vi "CalculateLuhnNumber.vi"(10 "InputString":string) -> (2 "String 2":string, 4 "Valid":bool)   [LabVIEW 2022 SP3]
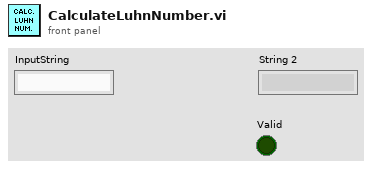
[diagram p1: front panel]
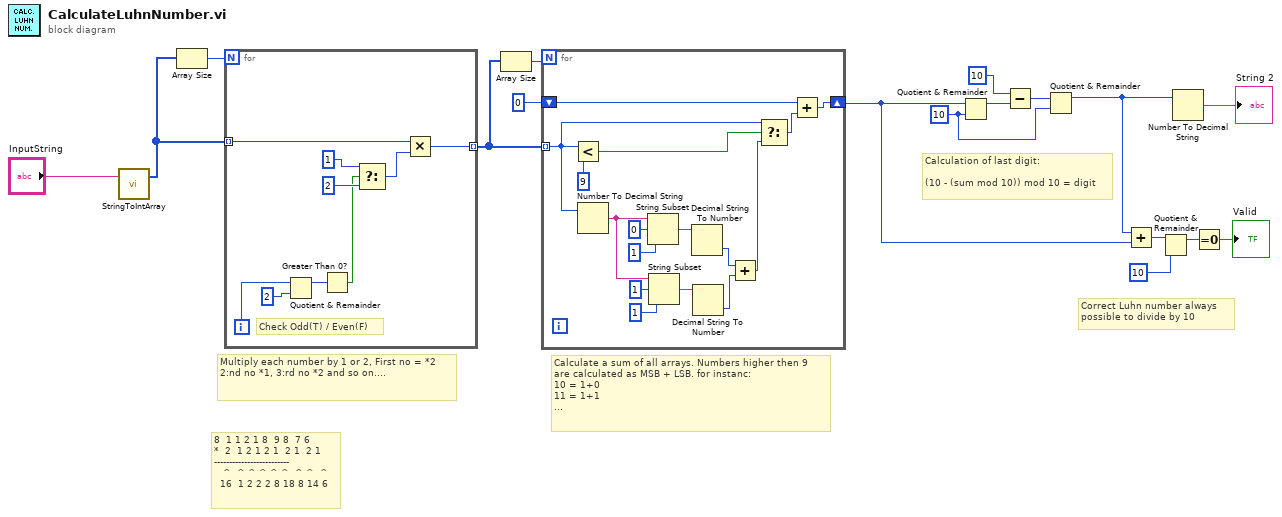
[diagram p0: block diagram]
diagram:
  w7 = 10 ("y")
  # "Correct Luhn number always\npossible to divide by 10"
  # "Calculation of last digit:\n\n(10 - (sum mod 10)) mod 10 = digit"
  # "8  1 1 2 1 8  9 8  7 6\n*  2  1 2 1 2 1  2 1  2 1\n-------------------------\n   ^  ^ ^ ^ ^ ^  ^ ^  ^ \n  16  1 2 2 2 8 18 8 14 6"
  # "Calculate a sum of all arrays. Numbers higher then 9\nare calculated as MSB + LSB. for instanc:\n10 = 1+0\n11 = 1+1\n..."
  # "Multiply each number by 1 or 2, First no = *2\n2:nd no *1, 3:rd no *2 and so on...."
  n1 = call "StringToIntArray.vi"("InputString"="InputString") -> ("OutArray"=w15:i32[])  [unwired: 1 in, 1 out]
  n2 = Array Size(array=w15) -> (size(s)=w16:i32)
  n3 = for {
    N: w16 -> [_]
    tunnel: w15 -> [w23] mode=indexing
    tunnel: [w18] -> w13 mode=indexing
    i -> [w24]
    # "Check Odd(T) / Even(F)"
    n4 = Quotient & Remainder(x=w24, y=2) -> (x-y*floor(x/y)=w26:i32)  [unwired: 1 out]
    n5 = Greater Than 0?(x=w26) -> (x > 0?=w19:bool)
    n6 = Select(t=1, s=w19, f=2) -> (s? t:f=w22:i32)
    n7 = Multiply(x=w23, y=w22) -> (x*y=w18:i32)
  }
  n8 = Array Size(array=w13) -> (size(s)=w14:i32)
  n9 = for {
    N: w14 -> [_]
    tunnel: w13 -> [w37] mode=indexing
    shift-right: [w41] -> w5
    shift-left: 0 -> [w39]
    n10 = Less?(x=w37, y=9) -> (x < y?=w40:bool)
    n11 = Number To Decimal String(number=w37) -> (decimal integer string=w30:string)  [unwired: 1 in]
    n12 = String Subset(string=w30, offset (0)=0, length (rest)=1 ("length (rest)")) -> (substring=w34:string)
    n13 = String Subset(string=w30, offset (0)=1, length (rest)=1 ("length (rest)")) -> (substring=w31:string)
    n14 = Decimal String To Number(string=w34) -> (number=w29:i32)  [unwired: 2 in, 1 out]
    n15 = Decimal String To Number(string=w31) -> (number=w28:i32)  [unwired: 2 in, 1 out]
    n16 = Add(x=w29, y=w28) -> (x+y=w27:i32)
    n17 = Select(t=w37, s=w40, f=w27) -> (s? t:f=w38:i32)
    n18 = Add(x=w39, y=w38) -> (x+y=w41:i32)
  }
  n19 = Quotient & Remainder(x=w5, y=w7) -> (x-y*floor(x/y)=w11:i32)  [unwired: 1 out]
  n20 = Subtract(x=10, y=w11) -> (x-y=w9:i32)
  n21 = Quotient & Remainder(x=w9, y=w7) -> (x-y*floor(x/y)=w6:i32)  [unwired: 1 out]
  n22 = Add(x=w6, y=w5) -> (x+y=w4:i32)
  n23 = Quotient & Remainder(x=w4, y=10) -> (x-y*floor(x/y)=w2:i32)  [unwired: 1 out]
  n24 = Number To Decimal String(number=w6) -> (decimal integer string=→"String 2":string)  [unwired: 1 in]
  n25 = Equal To 0?(x=w2) -> (x = 0?=→"Valid":bool)
